vi "GuiderSetupGUI.vi"() -> ()   [LabVIEW 2018]
uses:
  GuiderSetup/GuiderSetup.lvclass
  C:/Users/devstaff/sparc4/s4gui/Versao ZeroMQ REQ-REP/SPARC4_GUI -v1.0.8 - reconhecimento do ACK do ACS/S4GUI/S4GUI.lvclass
  S4GUI/S4GUI.lvclass/S4GUI.ctl
  Instrument/Instrument.lvclass/Instrument.ctl
  Device/Optics/Optics.lvclass/Optics.ctl
  Device/Optics/Opt_Continuous/Opt_Continuous.lvclass
  C:/Users/devstaff/sparc4/s4gui/Versao ZeroMQ REQ-REP/SPARC4_GUI -v1.0.8 - reconhecimento do ACK do ACS/Device/Optics/Optics.lvclass
  Instrument/Instrument.lvclass
  AG/AG.lvclass
  Device/angles/angles.lvclass
  S4GUI/S4GUI.lvclass
  Device/Optics/Optics.lvclass
  StateMachine/State Machine.lvclass
panel:
  out "GUI version":string
  in  "Tab Focus":enum32{"FOCUS", "Config"}(tab)
  in  "Guider Focus Target":dbl caption="Target" min=0.0 max=24.9 step=0.1
  in  "GOTO GFOC":bool
  in  "STOP GFOC":bool
  in  "GFOC IN":bool
  in  "GFOC OUT":bool
  out "Pos GFOC":dbl caption="Position (mm)" format="%3_4g"
  out "GFOC status":bool
  in  "Guider Focus Incr":dbl caption="Increment" min=0.0 max=5.0 step=0.01 format="%#2_4g"
  in  "Set Focus by Mode":bool
  in  "Focus by Mode":T1={"Phot."=17.0, "Polarim"=7.0, "Efficiency"=0.0, "Instrumental"=0.0}
  out "AG connection":bool caption="AG"
  in  "Rotator":dbl caption="ROTATOR"
  out "loop max (ms)":u32
  out "loop time (ms)":u32
  in  "Guider Mirror Veloc":dbl=1.0 caption="Veloc. (1-30)" min=1.0 max=30.0 step=1.0
  out "GMIR status":bool
  out "ICS connection":bool caption="ICS"
  out "error out":errorcluster
  out "Pos GMIR":dbl caption="Position (deg)" format="%-3_4g"
  in  "RUN GMIR":bool
  in  "STOP GMIR":bool
  in  "GOTO GMIR":bool
  in  "Guider Mirror Target":dbl caption="Target"
  in  "stop":bool
  in  "GuiderSetup.lvclass":refnum<class "GuiderSetup.lvclass">
  # "GUIDER SETUP"
  # "MIRROR"
  # "deg"
  # "deg/s"
  # "FOCUS"
  # "mm"
  # "mm"
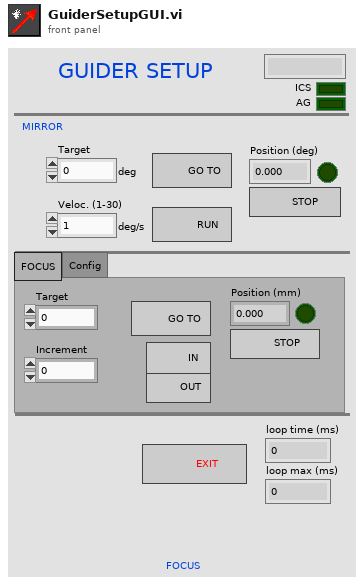
[diagram p1: front panel]
types:
  T1 = cluster{"Phot.":dbl, "Polarim":dbl, "Efficiency":dbl, "Instrumental":dbl}
  T2 = cluster{"Trigger Mode Status":string, "String output":string, "Instrument Status":cluster{"WPROT pos":dbl, "WPSEL pos":dbl, "GMIR pos":dbl, "GFOC pos":dbl, "CALW pos":dbl, "ASEL pos":dbl, "mode":bool, "String Status":string, "connection":bool, "operational":bool}, "Sync Box State":i32, "Trigger General Status":string, "Instrument States":cluster{"WPSEL State":i32, "WPROT State":i32, "CALW State":i32, "ASEL State":i32, "GMIR State":i32, "GFOC State":i32}, "Instrument Pos Names":cluster{"WPROT posname":string, "WPSEL posname":string, "CALW posname":string, "ASEL posname":string}, "ChannelA_Status":cluster{"Current exp":dbl, "Frames done":u32, "LastFileImage":string, "CamStatus":string, "Run state":u32, "connection":bool, "Cooler ON/OFF":i16, "Currently temperature":i16, "Temperature Status":string, "target  temp":i16, "conf runing":bool, "FT":bool, "UsedDisk":u16, "operational":bool}, "WPROT seq":u16, "ChannelB_Status":cluster{"Current exp":dbl, "Frames done":u32, "LastFileImage":string, "CamStatus":string, "Run state":u32, "connection":bool, "Cooler ON/OFF":i16, "Currently temperature":i16, "Temperature Status":string, "target  temp":i16, "conf runing":bool, "FT":bool, "UsedDisk":u16, "operational":bool}, "ChannelC_Status":cluster{"Current exp":dbl, "Frames done":u32, "LastFileImage":string, "CamStatus":string, "Run state":u32, "connection":bool, "Cooler ON/OFF":i16, "Currently temperature":i16, "Temperature Status":string, "target  temp":i16, "conf runing":bool, "FT":bool, "UsedDisk":u16, "operational":bool}, "ChannelD_Status":cluster{"Current exp":dbl, "Frames done":u32, "LastFileImage":string, "CamStatus":string, "Run state":u32, "connection":bool, "Cooler ON/OFF":i16, "Currently temperature":i16, "Temperature Status":string, "target  temp":i16, "conf runing":bool, "FT":bool, "UsedDisk":u16, "operational":bool}, "ChannelA_CCD":cluster{"ACQUISITION_MODE":u8, "TRIGGER_MODE":u8, "READ_MODE":u8, "PREAMP":u8, "READOUT_RATE":u8, "VERTICAL_SHIFT_SPEED":u8, "EM_MODE":u8, "EM_GAIN":u16, "SHUTTER_MODE":u8, "SHUTTER_TTL":u8, "SHUTTER_OPENNING_TIME":u16, "SHUTTER_CLOSING_TIME":u16, "VBIN":u16, "HBIN":u16, "INITIAL_LINE":u16, "INITIAL_COLUMN":u16, "FINAL_LINE":u16, "FINAL_COLUMN":u16, "FRAME_TRANSFER":bool, "VERTICAL_CLOCK_VOLTAGE":u8, "AD_CHANNEL":u32}, "ChannelB_CCD ":cluster{"ACQUISITION_MODE":u8, "TRIGGER_MODE":u8, "READ_MODE":u8, "PREAMP":u8, "READOUT_RATE":u8, "VERTICAL_SHIFT_SPEED":u8, "EM_MODE":u8, "EM_GAIN":u16, "SHUTTER_MODE":u8, "SHUTTER_TTL":u8, "SHUTTER_OPENNING_TIME":u16, "SHUTTER_CLOSING_TIME":u16, "VBIN":u16, "HBIN":u16, "INITIAL_LINE":u16, "INITIAL_COLUMN":u16, "FINAL_LINE":u16, "FINAL_COLUMN":u16, "FRAME_TRANSFER":bool, "VERTICAL_CLOCK_VOLTAGE":u8, "AD_CHANNEL":u32}, "ChannelC_CCD":cluster{"ACQUISITION_MODE":u8, "TRIGGER_MODE":u8, "READ_MODE":u8, "PREAMP":u8, "READOUT_RATE":u8, "VERTICAL_SHIFT_SPEED":u8, "EM_MODE":u8, "EM_GAIN":u16, "SHUTTER_MODE":u8, "SHUTTER_TTL":u8, "SHUTTER_OPENNING_TIME":u16, "SHUTTER_CLOSING_TIME":u16, "VBIN":u16, "HBIN":u16, "INITIAL_LINE":u16, "INITIAL_COLUMN":u16, "FINAL_LINE":u16, "FINAL_COLUMN":u16, "FRAME_TRANSFER":bool, "VERTICAL_CLOCK_VOLTAGE":u8, "AD_CHANNEL":u32}, "ChannelD_CCD":cluster{"ACQUISITION_MODE":u8, "TRIGGER_MODE":u8, "READ_MODE":u8, "PREAMP":u8, "READOUT_RATE":u8, "VERTICAL_SHIFT_SPEED":u8, "EM_MODE":u8, "EM_GAIN":u16, "SHUTTER_MODE":u8, "SHUTTER_TTL":u8, "SHUTTER_OPENNING_TIME":u16, "SHUTTER_CLOSING_TIME":u16, "VBIN":u16, "HBIN":u16, "INITIAL_LINE":u16, "INITIAL_COLUMN":u16, "FINAL_LINE":u16, "FINAL_COLUMN":u16, "FRAME_TRANSFER":bool, "VERTICAL_CLOCK_VOLTAGE":u8, "AD_CHANNEL":u32}, "CHA_Checked Params":cluster{"ACQUISITION_MODE":bool, "TRIGGER_MODE":bool, "READ_MODE":bool, "PREAMP":bool, "READOUT_RATE":bool, "VERTICAL_SHIFT_SPEED":bool, "EM_MODE":bool, "EM_GAIN":bool, "SHUTTER_MODE":bool, "SHUTTER_TTL":bool, "SHUTTER_OPENING_TIME":bool, "SHUTTER_CLOSING_TIME":bool, "VBIN":bool, "HBIN":bool, "INITIAL_LINE":bool, "INITIAL_COLUMN":bool, "FINAL_LINE":bool, "FINAL_COLUMN":bool, "FRAME_TRANSFER":bool, "VERTICAL_CLOCK_VOLTAGE":bool, "AD_CHANNEL":bool}, "CHB_Checked Params":cluster{"ACQUISITION_MODE":bool, "TRIGGER_MODE":bool, "READ_MODE":bool, "PREAMP":bool, "READOUT_RATE":bool, "VERTICAL_SHIFT_SPEED":bool, "EM_MODE":bool, "EM_GAIN":bool, "SHUTTER_MODE":bool, "SHUTTER_TTL":bool, "SHUTTER_OPENING_TIME":bool, "SHUTTER_CLOSING_TIME":bool, "VBIN":bool, "HBIN":bool, "INITIAL_LINE":bool, "INITIAL_COLUMN":bool, "FINAL_LINE":bool, "FINAL_COLUMN":bool, "FRAME_TRANSFER":bool, "VERTICAL_CLOCK_VOLTAGE":bool, "AD_CHANNEL":bool}, "CHC_Checked Params":cluster{"ACQUISITION_MODE":bool, "TRIGGER_MODE":bool, "READ_MODE":bool, "PREAMP":bool, "READOUT_RATE":bool, "VERTICAL_SHIFT_SPEED":bool, "EM_MODE":bool, "EM_GAIN":bool, "SHUTTER_MODE":bool, "SHUTTER_TTL":bool, "SHUTTER_OPENING_TIME":bool, "SHUTTER_CLOSING_TIME":bool, "VBIN":bool, "HBIN":bool, "INITIAL_LINE":bool, "INITIAL_COLUMN":bool, "FINAL_LINE":bool, "FINAL_COLUMN":bool, "FRAME_TRANSFER":bool, "VERTICAL_CLOCK_VOLTAGE":bool, "AD_CHANNEL":bool}, "CHD_Checked Params":cluster{"ACQUISITION_MODE":bool, "TRIGGER_MODE":bool, "READ_MODE":bool, "PREAMP":bool, "READOUT_RATE":bool, "VERTICAL_SHIFT_SPEED":bool, "EM_MODE":bool, "EM_GAIN":bool, "SHUTTER_MODE":bool, "SHUTTER_TTL":bool, "SHUTTER_OPENING_TIME":bool, "SHUTTER_CLOSING_TIME":bool, "VBIN":bool, "HBIN":bool, "INITIAL_LINE":bool, "INITIAL_COLUMN":bool, "FINAL_LINE":bool, "FINAL_COLUMN":bool, "FRAME_TRANSFER":bool, "VERTICAL_CLOCK_VOLTAGE":bool, "AD_CHANNEL":bool}, "Trigger_connection":bool, "TCSPD_connection":bool, "TCS extended":string, "TCS id":u32, "S4ICS id":u32, "focus pos":i32, "Focus_connection":bool, "WS_connection":bool, "weather status":cluster{"broker":string, "version":string, "date":string, "hour":string, "outHumidity":string, "inHumidity":string, "inTemp":string, "outTemp":string, "windSpeed":string, "windDirection":string, "pressure":string, "dewOut":string, "dewIn":string, "leaf":string, "rain":string, "windChill":string}, "GS STATUS cluster":cluster{"FocusPhot":dbl, "FocusPolar":dbl, "FocusEffic":dbl, "FocusInstrum":dbl, "ICS":bool, "AG":bool, "BROKER":string, "timestamp":string, "FocusPos":dbl, "MirrorPos":dbl}, "TCSPD_operational":bool, "Focus_operational":bool, "object_suffix":string, "dflat_suffix":string, "sflat_suffix":string, "dark_suffix":string, "zero_suffix":string, "focus_suffix":string, "suffixAlertVisible":bool, "Instrument Motor error":cluster{"WPSEL error":bool, "WPROT error":bool, "CALW error":bool, "ASEL error":bool, "GMIR error":bool, "GFOC error":bool}}
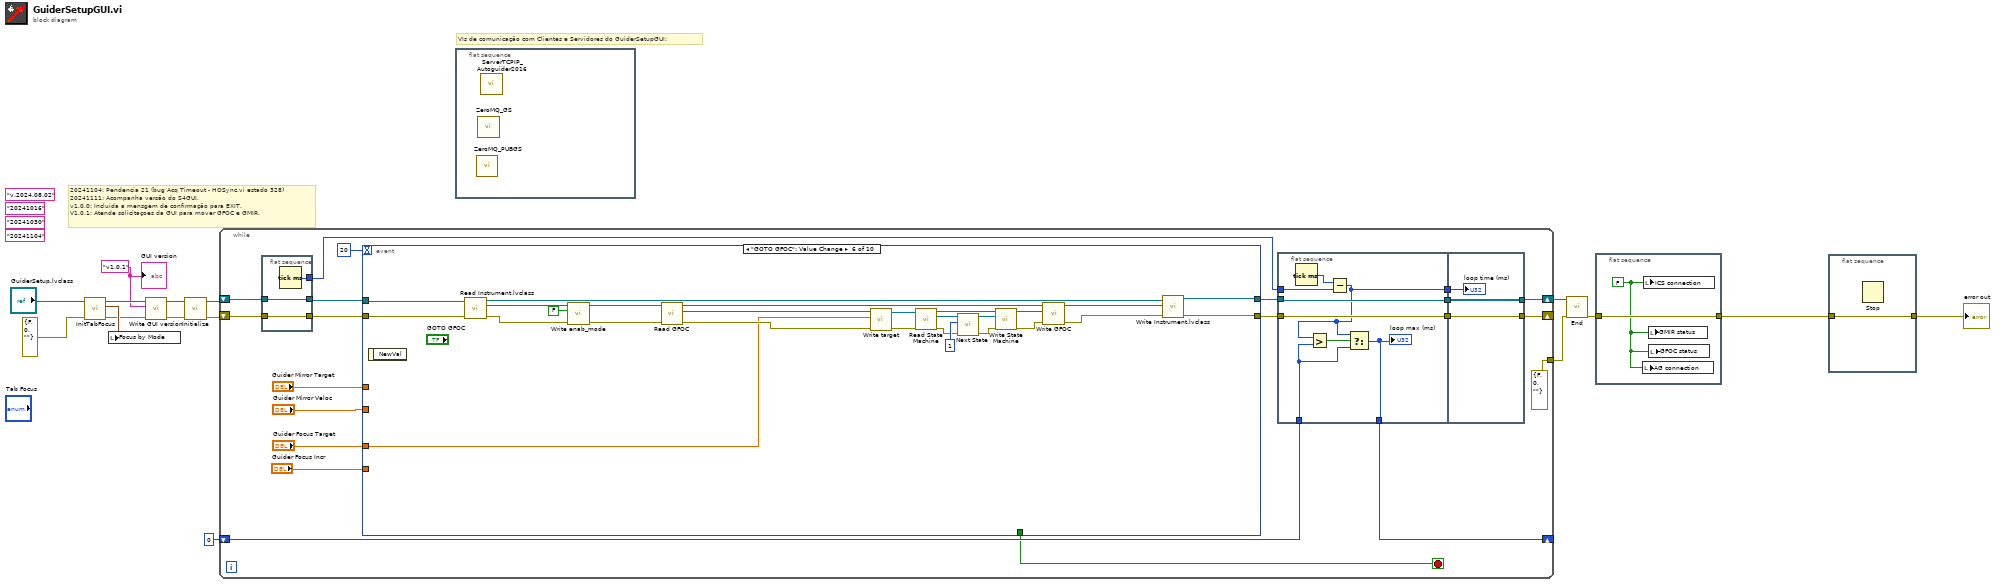
[diagram p0: block diagram]
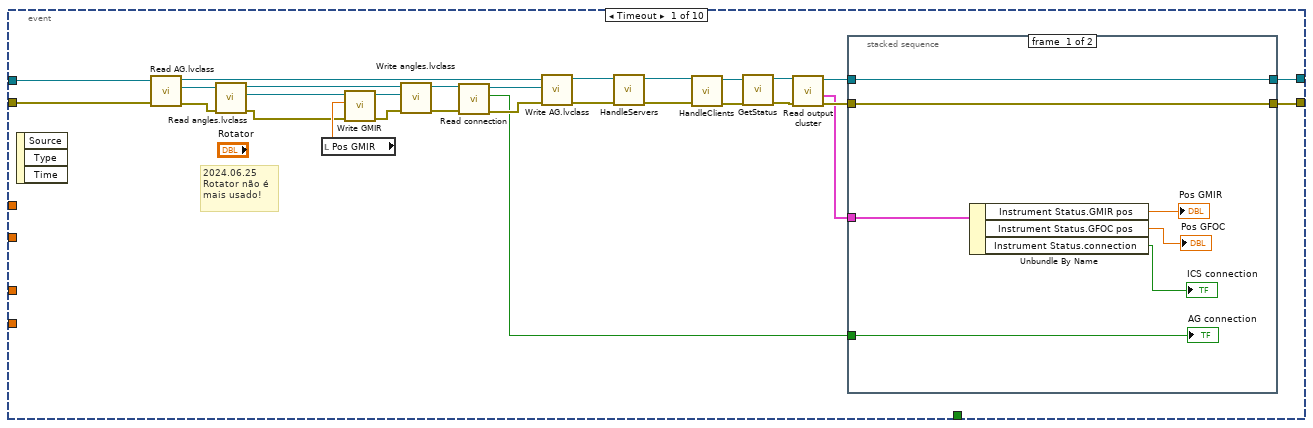
[diagram p2: hidden frame]
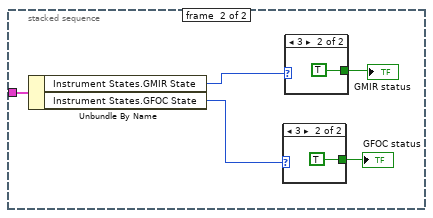
[diagram p3: hidden frame]
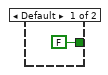
[diagram p4: hidden frame]
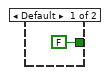
[diagram p5: hidden frame]
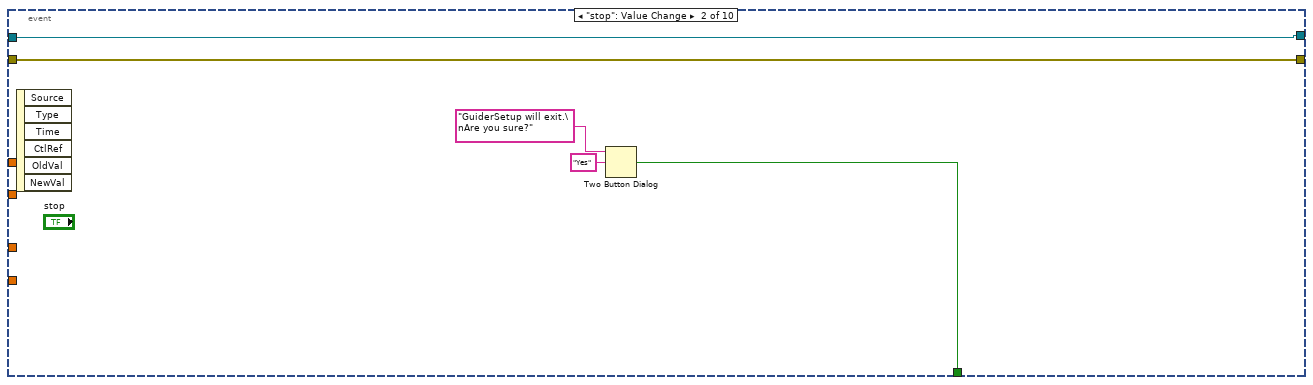
[diagram p6: hidden frame]
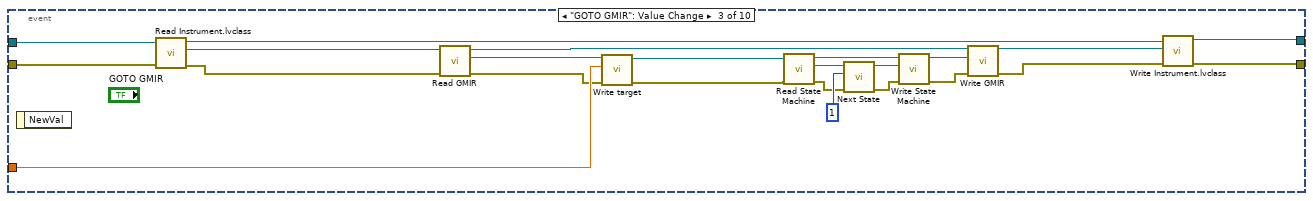
[diagram p7: hidden frame]
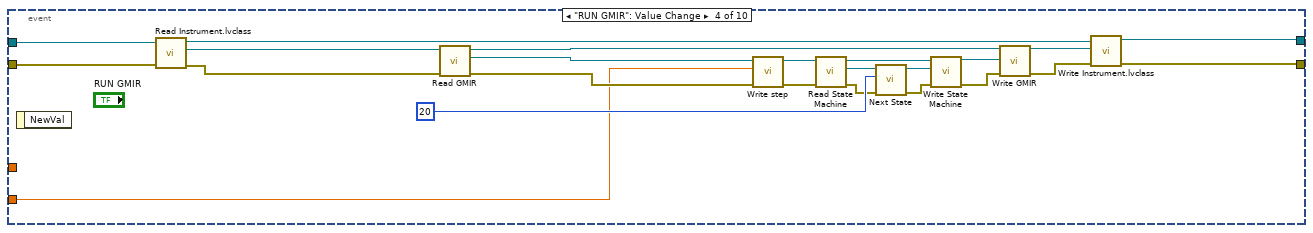
[diagram p8: hidden frame]
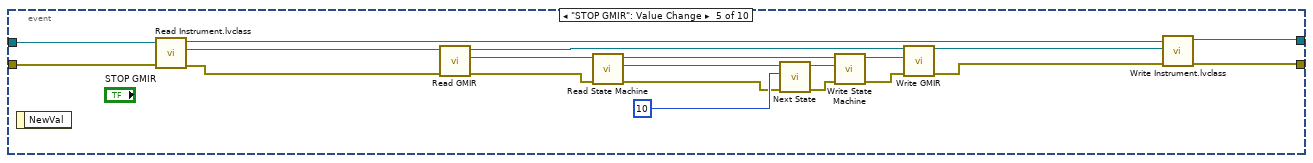
[diagram p9: hidden frame]
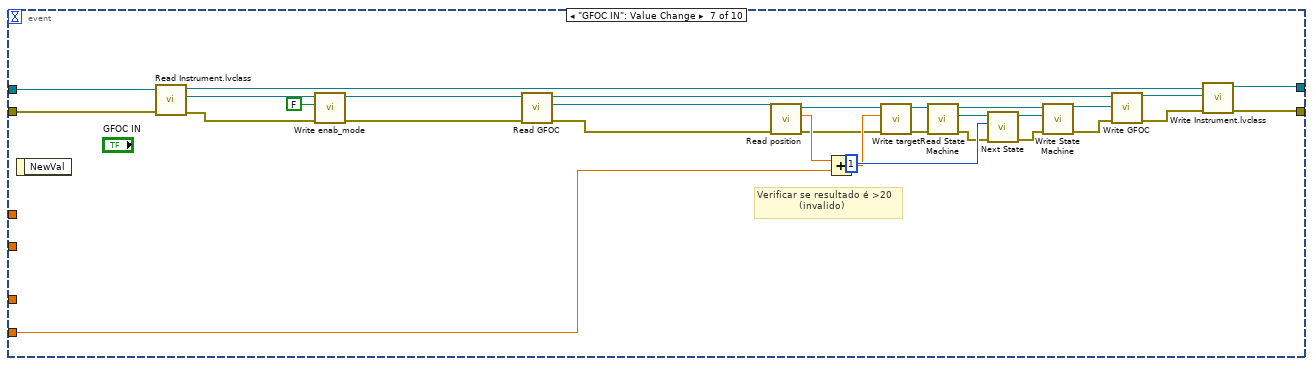
[diagram p10: hidden frame]
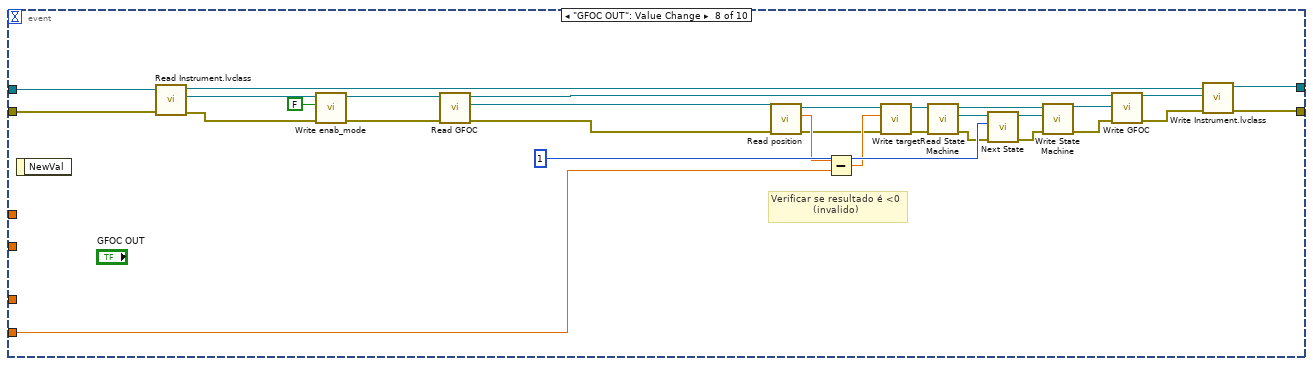
[diagram p11: hidden frame]
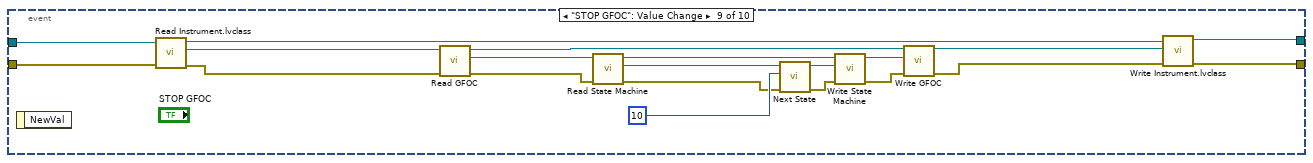
[diagram p12: hidden frame]
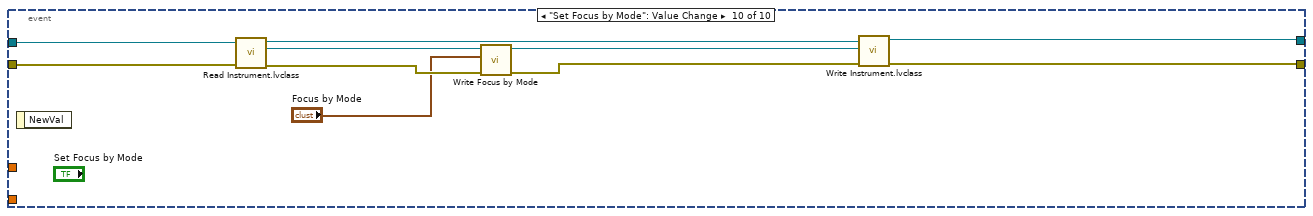
[diagram p13: hidden frame]
diagram:
  (unwired) "20241104" ("GUI version")
  (unwired) "20241030" ("GUI version")
  (unwired) "20241016" ("GUI version")
  w1 = "v1.0.1" ("GUI version")
  (unwired) "v.2024.08.02" ("GUI version")
  # "20241104: Pendencia 21 (bug Acq Timeout - HOSync.vi estado 328)\n20241111: Acompanha versão do S4GUI.\nv1.0.0: Incluída a mensgem de confirmação para EXIT.\nV1.0.1: Atende solicitaçoes da GUI para mover GFOC e GMIR."
  # "VIs de comunicação com Clientes e Servidores do GuiderSetupGUI:"
  n1 = call-dynamic "InitTabFocus.vi"("error in (no error)"=errorcluster {"status"=FALSE, "code"=0, "source"=""}, "GuiderSetup in"="GuiderSetup.lvclass") -> ("error out"=w5:errorcluster, "output cluster"=w8:T1, "GuiderSetup out"=w7:refnum<class "GuiderSetup.lvclass">)  [unwired: 7 in]
  n2 = local write "Focus by Mode"(w8) -> ()
  n3 = call-dynamic "Write GUI version.vi"("error in (no error)"=w5, "GUI version"=w1, "S4GUI in"=w7) -> ("error out"=w4:errorcluster, "S4GUI out"=w6:refnum<class "GuiderSetup.lvclass">)  [unwired: 7 in]
  n4 = call-dynamic "Initialize.vi"("error in (no error)"=w4, "S4ACS_GUI in"=w6) -> ("error out"=w15:errorcluster, "S4ACS_GUI out"=w16:refnum<class "GuiderSetup.lvclass">)  [unwired: 8 in]
  n5 = while {
    shift-right: [w25] -> w14
    shift-left: w16 -> [w32]
    shift-right: [w26] -> _
    shift-left: w15 -> [w31]
    shift-right: [w20] -> _
    shift-left: u32 0 -> [w19]
    tunnel: [errorcluster {"status"=FALSE, "code"=0, "source"=""} ("error in (no error)")] -> w11
    stop <- w17 stop-if-true
    n6 = flat-sequence {
      tunnel: [w51] -> w21
      tunnel: w32 -> [w50]
      tunnel: w31 -> [w49]
      tunnel: [w50] -> w30
      tunnel: [w49] -> w29
      frame #0 {
        n7 = Tick Count (ms)() -> (millisecond timer value=w51:u32)
      }
    }
    n8 = event shown="[5] \"GOTO GFOC\": Value Change" {
      selector: _ -> [_ _ _ _ _ _ _ _ _ _]
      dyn-events: _ -> [_ _ _ _ _ _ _ _ _ _]
      timeout: 20 -> [_ _ _ _ _ _ _ _ _ _]
      tunnel: w30 -> [w80 w101 w124 w147 w167 w193 w223 w253 w273 w283]
      tunnel: [w64 w101 w122 w145 w165 w191 w221 w251 w271 w281] -> w28
      tunnel: w29 -> [w79 w98 w118 w141 w161 w188 w218 w248 w267 w280]
      tunnel: [w61 w98 w115 w138 w158 w186 w216 w246 w264 w279] -> w27
      tunnel: "Guider Mirror Veloc" -> [_ _ _ w125 _ _ _ _ _ _]
      tunnel: "Guider Mirror Target" -> [_ _ w104 _ _ _ _ _ _ _]
      tunnel: "Guider Focus Target" -> [_ _ _ _ _ w173 _ _ _ _]
      tunnel: "Guider Focus Incr" -> [_ _ _ _ _ _ w199 w229 _ _]
      tunnel: [_ w99 _ _ _ _ _ _ _ _] -> w17
      event Timeout {
        # "2024.06.25\nRotator não é \nmais usado!"
        n9 = event-data() -> ()  [unwired: 1 in, 3 out]
        n10 = call-dynamic "Read AG.lvclass.vi"("error in (no error)"=w79, "GuiderSetup in"=w80) -> ("error out"=w74:errorcluster, "AG.lvclass"=w77:refnum<class "AG.lvclass">, "GuiderSetup out"=w78:refnum<class "GuiderSetup.lvclass">)  [unwired: 7 in]
        n11 = call-dynamic "Read angles.lvclass.vi"("error in (no error)"=w74, "AG in"=w77) -> ("error out"=w62:errorcluster, "angles.lvclass"=w63:refnum<class "angles.lvclass">, "AG out"=w76:refnum<class "AG.lvclass">)  [unwired: 7 in]
        n12 = local read "Pos GMIR"() -> (w72:dbl)
        n13 = call-dynamic "Write GMIR.vi"("error in (no error)"=w62, "GMIR"=w72, "angles in"=w63) -> ("error out"=w73:errorcluster, "angles out"=w75:refnum<class "angles.lvclass">)  [unwired: 7 in]
        n14 = call-dynamic "Write angles.lvclass.vi"("error in (no error)"=w73, "angles.lvclass"=w75, "AG in"=w76) -> ("error out"=w67:errorcluster, "AG out"=w69:refnum<class "AG.lvclass">)  [unwired: 7 in]
        n15 = call-dynamic "Read connection.vi"("error in (no error)"=w67, "Client in"=w69) -> ("error out"=w66:errorcluster, "connection"=w65:bool, "Client out"=w68:refnum<class "AG.lvclass">)  [unwired: 7 in]
        n16 = call-dynamic "Write AG.lvclass.vi"("error in (no error)"=w66, "AG.lvclass"=w68, "GuiderSetup in"=w78) -> ("error out"=w71:errorcluster, "GuiderSetup out"=w70:refnum<class "GuiderSetup.lvclass">)  [unwired: 7 in]
        n17 = call-dynamic "HandleServers.vi"("error in (no error)"=w71, "S4ACS_GUI in"=w70) -> ("error out"=w58:errorcluster, "S4ACS_GUI out"=w60:refnum<class "GuiderSetup.lvclass">)  [unwired: 8 in]
        n18 = call-dynamic "HandleClients.vi"("error in (no error)"=w58, "GuiderSetup in"=w60) -> ("error out"=w57:errorcluster, "GuiderSetup out"=w59:refnum<class "GuiderSetup.lvclass">)  [unwired: 8 in]
        n19 = call-dynamic "GetStatus.vi"("error in (no error)"=w57, "GS in"=w59) -> ("error out"=w54:errorcluster, "GS out"=w56:refnum<class "GuiderSetup.lvclass">)  [unwired: 8 in]
        n20 = call-dynamic "Read output cluster.vi"("error in (no error)"=w54, "S4GUI in"=w56) -> ("error out"=w53:errorcluster, "output cluster"=w52:T2, "S4GUI out"=w55:refnum<class "GuiderSetup.lvclass">)  [unwired: 7 in]
        n21 = stacked-sequence {
          tunnel: w65 -> [w84 _]
          tunnel: w55 -> [w83 _]
          tunnel: w53 -> [w82 _]
          tunnel: [w83 _] -> w64
          tunnel: [w82 _] -> w61
          tunnel: w52 -> [w81 w88]
          frame #0 {
            n22 = Unbundle By Name(w81) -> ("Instrument Status.GMIR pos"=→"Pos GMIR":dbl, "Instrument Status.GFOC pos"=→"Pos GFOC":dbl, "Instrument Status.connection"=→"ICS connection":bool)
            "AG connection" <- w84
          }
          frame #1 {
            n23 = Unbundle By Name(w88) -> ("Instrument States.GMIR State"=w92:i32, "Instrument States.GFOC State"=w90:i32)
            n24 = case shown="3" w90 {
              tunnel: [FALSE TRUE] -> w89
              frame Default {
              }
              frame 3 {
              }
            }
            "GFOC status" <- w89
            n25 = case shown="3" w92 {
              tunnel: [FALSE TRUE] -> w91
              frame Default {
              }
              frame 3 {
              }
            }
            "GMIR status" <- w91
          }
        }
      }
      event "stop": Value Change {
        n26 = event-data() -> ()  [unwired: 1 in, 6 out]
        n27 = Two Button Dialog(message="GuiderSetup will exit.\nAre you sure?", 2:"Yes" ("T button name (\"OK\")")) -> (T button?=w99:bool)  [unwired: 1 in]
      }
      event "GOTO GMIR": Value Change {
        n28 = event-data() -> ()  [unwired: 1 in, 1 out]
        n29 = call "Read Instrument.lvclass.vi"("error in (no error)"=w118, "S4ACS_GUI in"=w124) -> ("error out"=w117:errorcluster, "Instrument.lvclass"=w121:refnum<class "Instrument.lvclass">, "S4ACS_GUI out"=w123:refnum<class "GuiderSetup.lvclass">)  [unwired: 7 in]
        n30 = call "Read GMIR.vi"("error in (no error)"=w117, "Instrument in"=w121) -> ("error out"=w103:errorcluster, "Opt_Continuous.lvclass"=w106:refnum<class "Opt_Continuous.lvclass">, "Instrument out"=w120:refnum<class "Instrument.lvclass">)  [unwired: 7 in]
        n31 = call "Write target.vi"("error in (no error)"=w103, "target"=w104, "Optics in"=w106) -> ("error out"=w102:errorcluster, "Optics out"=w105:refnum<class "Opt_Continuous.lvclass">)  [unwired: 7 in]
        n32 = call-dynamic "Read State Machine.vi"("error in (no error)"=w102, "Device in"=w105) -> ("error out"=w109:errorcluster, "State Machine.lvclass"=w112:refnum<class "State Machine.lvclass">, "Device out"=w114:refnum<class "Opt_Continuous.lvclass">)  [unwired: 7 in]
        n33 = call "Next State.vi"("error in (no error)"=w109, "New_State"=1, "State Machine in"=w112) -> ("error out"=w108:errorcluster, "State Machine out"=w111:refnum<class "State Machine.lvclass">)  [unwired: 7 in]
        n34 = call-dynamic "Write State Machine.vi"("error in (no error)"=w108, "State Machine.lvclass"=w111, "Device in"=w114) -> ("error out"=w107:errorcluster, "Device out"=w113:refnum<class "Opt_Continuous.lvclass">)  [unwired: 7 in]
        n35 = call "Write GMIR.vi"("error in (no error)"=w107, "Opt_Continuous.lvclass"=w113, "Instrument in"=w120) -> ("error out"=w116:errorcluster, "Instrument out"=w119:refnum<class "Instrument.lvclass">)  [unwired: 7 in]
        n36 = call "Write Instrument.lvclass.vi"("error in (no error)"=w116, "Instrument.lvclass"=w119, "S4ACS_GUI in"=w123) -> ("error out"=w115:errorcluster, "S4ACS_GUI out"=w122:refnum<class "GuiderSetup.lvclass">)  [unwired: 7 in]
      }
      event "RUN GMIR": Value Change {
        n37 = event-data() -> ()  [unwired: 1 in, 1 out]
        n38 = call "Read Instrument.lvclass.vi"("error in (no error)"=w141, "S4ACS_GUI in"=w147) -> ("error out"=w140:errorcluster, "Instrument.lvclass"=w144:refnum<class "Instrument.lvclass">, "S4ACS_GUI out"=w146:refnum<class "GuiderSetup.lvclass">)  [unwired: 7 in]
        n39 = call "Read GMIR.vi"("error in (no error)"=w140, "Instrument in"=w144) -> ("error out"=w128:errorcluster, "Opt_Continuous.lvclass"=w129:refnum<class "Opt_Continuous.lvclass">, "Instrument out"=w143:refnum<class "Instrument.lvclass">)  [unwired: 7 in]
        n40 = call-dynamic "Write step.vi"("error in (no error)"=w128, "step"=w125, "Optics in"=w129) -> ("error out"=w127:errorcluster, "Optics out"=w126:refnum<class "Opt_Continuous.lvclass">)  [unwired: 7 in]
        n41 = call-dynamic "Read State Machine.vi"("error in (no error)"=w127, "Device in"=w126) -> ("error out"=w132:errorcluster, "State Machine.lvclass"=w135:refnum<class "State Machine.lvclass">, "Device out"=w137:refnum<class "Opt_Continuous.lvclass">)  [unwired: 7 in]
        n42 = call "Next State.vi"("error in (no error)"=w132, "New_State"=20, "State Machine in"=w135) -> ("error out"=w131:errorcluster, "State Machine out"=w134:refnum<class "State Machine.lvclass">)  [unwired: 7 in]
        n43 = call-dynamic "Write State Machine.vi"("error in (no error)"=w131, "State Machine.lvclass"=w134, "Device in"=w137) -> ("error out"=w130:errorcluster, "Device out"=w136:refnum<class "Opt_Continuous.lvclass">)  [unwired: 7 in]
        n44 = call "Write GMIR.vi"("error in (no error)"=w130, "Opt_Continuous.lvclass"=w136, "Instrument in"=w143) -> ("error out"=w139:errorcluster, "Instrument out"=w142:refnum<class "Instrument.lvclass">)  [unwired: 7 in]
        n45 = call "Write Instrument.lvclass.vi"("error in (no error)"=w139, "Instrument.lvclass"=w142, "S4ACS_GUI in"=w146) -> ("error out"=w138:errorcluster, "S4ACS_GUI out"=w145:refnum<class "GuiderSetup.lvclass">)  [unwired: 7 in]
      }
      event "STOP GMIR": Value Change {
        n46 = event-data() -> ()  [unwired: 1 in, 1 out]
        n47 = call "Read Instrument.lvclass.vi"("error in (no error)"=w161, "S4ACS_GUI in"=w167) -> ("error out"=w160:errorcluster, "Instrument.lvclass"=w164:refnum<class "Instrument.lvclass">, "S4ACS_GUI out"=w166:refnum<class "GuiderSetup.lvclass">)  [unwired: 7 in]
        n48 = call "Read GMIR.vi"("error in (no error)"=w160, "Instrument in"=w164) -> ("error out"=w151:errorcluster, "Opt_Continuous.lvclass"=w157:refnum<class "Opt_Continuous.lvclass">, "Instrument out"=w163:refnum<class "Instrument.lvclass">)  [unwired: 7 in]
        n49 = call-dynamic "Read State Machine.vi"("error in (no error)"=w151, "Device in"=w157) -> ("error out"=w150:errorcluster, "State Machine.lvclass"=w154:refnum<class "State Machine.lvclass">, "Device out"=w156:refnum<class "Opt_Continuous.lvclass">)  [unwired: 7 in]
        n50 = call "Next State.vi"("error in (no error)"=w150, "New_State"=10, "State Machine in"=w154) -> ("error out"=w149:errorcluster, "State Machine out"=w153:refnum<class "State Machine.lvclass">)  [unwired: 7 in]
        n51 = call-dynamic "Write State Machine.vi"("error in (no error)"=w149, "State Machine.lvclass"=w153, "Device in"=w156) -> ("error out"=w148:errorcluster, "Device out"=w155:refnum<class "Opt_Continuous.lvclass">)  [unwired: 7 in]
        n52 = call "Write GMIR.vi"("error in (no error)"=w148, "Opt_Continuous.lvclass"=w155, "Instrument in"=w163) -> ("error out"=w159:errorcluster, "Instrument out"=w162:refnum<class "Instrument.lvclass">)  [unwired: 7 in]
        n53 = call "Write Instrument.lvclass.vi"("error in (no error)"=w159, "Instrument.lvclass"=w162, "S4ACS_GUI in"=w166) -> ("error out"=w158:errorcluster, "S4ACS_GUI out"=w165:refnum<class "GuiderSetup.lvclass">)  [unwired: 7 in]
      }
      event "GOTO GFOC": Value Change {
        n54 = event-data() -> ()  [unwired: 1 in, 1 out]
        n55 = call "Read Instrument.lvclass.vi"("error in (no error)"=w188, "S4ACS_GUI in"=w193) -> ("error out"=w171:errorcluster, "Instrument.lvclass"=w172:refnum<class "Instrument.lvclass">, "S4ACS_GUI out"=w192:refnum<class "GuiderSetup.lvclass">)  [unwired: 7 in]
        n56 = call-dynamic "Write enab_mode.vi"("error in (no error)"=w171, "enab_mode"=FALSE, "Instrument in"=w172) -> ("error out"=w168:errorcluster, "Instrument out"=w169:refnum<class "Instrument.lvclass">)  [unwired: 7 in]
        n57 = call "Read GFOC.vi"("error in (no error)"=w168, "Instrument in"=w169) -> ("error out"=w175:errorcluster, "Opt_Continuous.lvclass"=w177:refnum<class "Opt_Continuous.lvclass">, "Instrument out"=w190:refnum<class "Instrument.lvclass">)  [unwired: 7 in]
        n58 = call "Write target.vi"("error in (no error)"=w175, "target"=w173, "Optics in"=w177) -> ("error out"=w174:errorcluster, "Optics out"=w176:refnum<class "Opt_Continuous.lvclass">)  [unwired: 7 in]
        n59 = call-dynamic "Read State Machine.vi"("error in (no error)"=w174, "Device in"=w176) -> ("error out"=w180:errorcluster, "State Machine.lvclass"=w183:refnum<class "State Machine.lvclass">, "Device out"=w185:refnum<class "Opt_Continuous.lvclass">)  [unwired: 7 in]
        n60 = call "Next State.vi"("error in (no error)"=w180, "New_State"=1, "State Machine in"=w183) -> ("error out"=w179:errorcluster, "State Machine out"=w182:refnum<class "State Machine.lvclass">)  [unwired: 7 in]
        n61 = call-dynamic "Write State Machine.vi"("error in (no error)"=w179, "State Machine.lvclass"=w182, "Device in"=w185) -> ("error out"=w178:errorcluster, "Device out"=w184:refnum<class "Opt_Continuous.lvclass">)  [unwired: 7 in]
        n62 = call "Write GFOC.vi"("error in (no error)"=w178, "Opt_Continuous.lvclass"=w184, "Instrument in"=w190) -> ("error out"=w187:errorcluster, "Instrument out"=w189:refnum<class "Instrument.lvclass">)  [unwired: 7 in]
        n63 = call "Write Instrument.lvclass.vi"("error in (no error)"=w187, "Instrument.lvclass"=w189, "S4ACS_GUI in"=w192) -> ("error out"=w186:errorcluster, "S4ACS_GUI out"=w191:refnum<class "GuiderSetup.lvclass">)  [unwired: 7 in]
      }
      event "GFOC IN": Value Change {
        # "Verificar se resultado é >20 \n              (invalido)"
        n64 = event-data() -> ()  [unwired: 1 in, 1 out]
        n65 = call "Read Instrument.lvclass.vi"("error in (no error)"=w218, "S4ACS_GUI in"=w223) -> ("error out"=w196:errorcluster, "Instrument.lvclass"=w197:refnum<class "Instrument.lvclass">, "S4ACS_GUI out"=w222:refnum<class "GuiderSetup.lvclass">)  [unwired: 7 in]
        n66 = call-dynamic "Write enab_mode.vi"("error in (no error)"=w196, "enab_mode"=FALSE, "Instrument in"=w197) -> ("error out"=w194:errorcluster, "Instrument out"=w195:refnum<class "Instrument.lvclass">)  [unwired: 7 in]
        n67 = call "Read GFOC.vi"("error in (no error)"=w194, "Instrument in"=w195) -> ("error out"=w200:errorcluster, "Opt_Continuous.lvclass"=w201:refnum<class "Opt_Continuous.lvclass">, "Instrument out"=w220:refnum<class "Instrument.lvclass">)  [unwired: 7 in]
        n68 = call "Read position.vi"("error in (no error)"=w200, "Optics in"=w201) -> ("error out"=w204:errorcluster, "position"=w207:dbl, "Optics out"=w205:refnum<class "Opt_Continuous.lvclass">)  [unwired: 7 in]
        n69 = Add(x=w207, y=w199) -> (x+y=w206:dbl)
        n70 = call "Write target.vi"("error in (no error)"=w204, "target"=w206, "Optics in"=w205) -> ("error out"=w203:errorcluster, "Optics out"=w202:refnum<class "Opt_Continuous.lvclass">)  [unwired: 7 in]
        n71 = call-dynamic "Read State Machine.vi"("error in (no error)"=w203, "Device in"=w202) -> ("error out"=w210:errorcluster, "State Machine.lvclass"=w213:refnum<class "State Machine.lvclass">, "Device out"=w215:refnum<class "Opt_Continuous.lvclass">)  [unwired: 7 in]
        n72 = call "Next State.vi"("error in (no error)"=w210, "New_State"=1, "State Machine in"=w213) -> ("error out"=w209:errorcluster, "State Machine out"=w212:refnum<class "State Machine.lvclass">)  [unwired: 7 in]
        n73 = call-dynamic "Write State Machine.vi"("error in (no error)"=w209, "State Machine.lvclass"=w212, "Device in"=w215) -> ("error out"=w208:errorcluster, "Device out"=w214:refnum<class "Opt_Continuous.lvclass">)  [unwired: 7 in]
        n74 = call "Write GFOC.vi"("error in (no error)"=w208, "Opt_Continuous.lvclass"=w214, "Instrument in"=w220) -> ("error out"=w217:errorcluster, "Instrument out"=w219:refnum<class "Instrument.lvclass">)  [unwired: 7 in]
        n75 = call "Write Instrument.lvclass.vi"("error in (no error)"=w217, "Instrument.lvclass"=w219, "S4ACS_GUI in"=w222) -> ("error out"=w216:errorcluster, "S4ACS_GUI out"=w221:refnum<class "GuiderSetup.lvclass">)  [unwired: 7 in]
      }
      event "GFOC OUT": Value Change {
        # "Verificar se resultado é <0\n              (invalido)"
        n76 = event-data() -> ()  [unwired: 1 in, 1 out]
        n77 = call "Read Instrument.lvclass.vi"("error in (no error)"=w248, "S4ACS_GUI in"=w253) -> ("error out"=w226:errorcluster, "Instrument.lvclass"=w227:refnum<class "Instrument.lvclass">, "S4ACS_GUI out"=w252:refnum<class "GuiderSetup.lvclass">)  [unwired: 7 in]
        n78 = call-dynamic "Write enab_mode.vi"("error in (no error)"=w226, "enab_mode"=FALSE, "Instrument in"=w227) -> ("error out"=w224:errorcluster, "Instrument out"=w225:refnum<class "Instrument.lvclass">)  [unwired: 7 in]
        n79 = call "Read GFOC.vi"("error in (no error)"=w224, "Instrument in"=w225) -> ("error out"=w230:errorcluster, "Opt_Continuous.lvclass"=w231:refnum<class "Opt_Continuous.lvclass">, "Instrument out"=w250:refnum<class "Instrument.lvclass">)  [unwired: 7 in]
        n80 = call "Read position.vi"("error in (no error)"=w230, "Optics in"=w231) -> ("error out"=w234:errorcluster, "position"=w237:dbl, "Optics out"=w235:refnum<class "Opt_Continuous.lvclass">)  [unwired: 7 in]
        n81 = Subtract(x=w237, y=w229) -> (x-y=w236:dbl)
        n82 = call "Write target.vi"("error in (no error)"=w234, "target"=w236, "Optics in"=w235) -> ("error out"=w233:errorcluster, "Optics out"=w232:refnum<class "Opt_Continuous.lvclass">)  [unwired: 7 in]
        n83 = call-dynamic "Read State Machine.vi"("error in (no error)"=w233, "Device in"=w232) -> ("error out"=w240:errorcluster, "State Machine.lvclass"=w243:refnum<class "State Machine.lvclass">, "Device out"=w245:refnum<class "Opt_Continuous.lvclass">)  [unwired: 7 in]
        n84 = call "Next State.vi"("error in (no error)"=w240, "New_State"=1, "State Machine in"=w243) -> ("error out"=w239:errorcluster, "State Machine out"=w242:refnum<class "State Machine.lvclass">)  [unwired: 7 in]
        n85 = call-dynamic "Write State Machine.vi"("error in (no error)"=w239, "State Machine.lvclass"=w242, "Device in"=w245) -> ("error out"=w238:errorcluster, "Device out"=w244:refnum<class "Opt_Continuous.lvclass">)  [unwired: 7 in]
        n86 = call "Write GFOC.vi"("error in (no error)"=w238, "Opt_Continuous.lvclass"=w244, "Instrument in"=w250) -> ("error out"=w247:errorcluster, "Instrument out"=w249:refnum<class "Instrument.lvclass">)  [unwired: 7 in]
        n87 = call "Write Instrument.lvclass.vi"("error in (no error)"=w247, "Instrument.lvclass"=w249, "S4ACS_GUI in"=w252) -> ("error out"=w246:errorcluster, "S4ACS_GUI out"=w251:refnum<class "GuiderSetup.lvclass">)  [unwired: 7 in]
      }
      event "STOP GFOC": Value Change {
        n88 = event-data() -> ()  [unwired: 1 in, 1 out]
        n89 = call "Read Instrument.lvclass.vi"("error in (no error)"=w267, "S4ACS_GUI in"=w273) -> ("error out"=w266:errorcluster, "Instrument.lvclass"=w270:refnum<class "Instrument.lvclass">, "S4ACS_GUI out"=w272:refnum<class "GuiderSetup.lvclass">)  [unwired: 7 in]
        n90 = call "Read GFOC.vi"("error in (no error)"=w266, "Instrument in"=w270) -> ("error out"=w257:errorcluster, "Opt_Continuous.lvclass"=w263:refnum<class "Opt_Continuous.lvclass">, "Instrument out"=w269:refnum<class "Instrument.lvclass">)  [unwired: 7 in]
        n91 = call-dynamic "Read State Machine.vi"("error in (no error)"=w257, "Device in"=w263) -> ("error out"=w256:errorcluster, "State Machine.lvclass"=w260:refnum<class "State Machine.lvclass">, "Device out"=w262:refnum<class "Opt_Continuous.lvclass">)  [unwired: 7 in]
        n92 = call "Next State.vi"("error in (no error)"=w256, "New_State"=10, "State Machine in"=w260) -> ("error out"=w255:errorcluster, "State Machine out"=w259:refnum<class "State Machine.lvclass">)  [unwired: 7 in]
        n93 = call-dynamic "Write State Machine.vi"("error in (no error)"=w255, "State Machine.lvclass"=w259, "Device in"=w262) -> ("error out"=w254:errorcluster, "Device out"=w261:refnum<class "Opt_Continuous.lvclass">)  [unwired: 7 in]
        n94 = call "Write GFOC.vi"("error in (no error)"=w254, "Opt_Continuous.lvclass"=w261, "Instrument in"=w269) -> ("error out"=w265:errorcluster, "Instrument out"=w268:refnum<class "Instrument.lvclass">)  [unwired: 7 in]
        n95 = call "Write Instrument.lvclass.vi"("error in (no error)"=w265, "Instrument.lvclass"=w268, "S4ACS_GUI in"=w272) -> ("error out"=w264:errorcluster, "S4ACS_GUI out"=w271:refnum<class "GuiderSetup.lvclass">)  [unwired: 7 in]
      }
      event "Set Focus by Mode": Value Change {
        n96 = event-data() -> ()  [unwired: 1 in, 1 out]
        n97 = call "Read Instrument.lvclass.vi"("error in (no error)"=w280, "S4ACS_GUI in"=w283) -> ("error out"=w277:errorcluster, "Instrument.lvclass"=w278:refnum<class "Instrument.lvclass">, "S4ACS_GUI out"=w282:refnum<class "GuiderSetup.lvclass">)  [unwired: 7 in]
        n98 = call-dynamic "Write Focus by Mode.vi"("error in (no error)"=w277, "Focus by Mode"="Focus by Mode", "Instrument in"=w278) -> ("error out"=w275:errorcluster, "Instrument out"=w276:refnum<class "Instrument.lvclass">)  [unwired: 7 in]
        n99 = call "Write Instrument.lvclass.vi"("error in (no error)"=w275, "Instrument.lvclass"=w276, "S4ACS_GUI in"=w282) -> ("error out"=w279:errorcluster, "S4ACS_GUI out"=w281:refnum<class "GuiderSetup.lvclass">)  [unwired: 7 in]
      }
    }
    n100 = flat-sequence {
      tunnel: w28 -> [w45]
      tunnel: w27 -> [w44]
      tunnel: w21 -> [w43]
      tunnel: [w45] -> w24
      tunnel: [w44] -> w23
      tunnel: [w40] -> w22
      tunnel: [w39] -> w20
      tunnel: w19 -> [w38]
      tunnel: [w47] -> w26
      tunnel: [w48] -> w25
      tunnel: w24 -> [w48]
      tunnel: w23 -> [w47]
      tunnel: w22 -> [w46]
      frame #0 {
        n101 = Tick Count (ms)() -> (millisecond timer value=w42:u32)
        n102 = Subtract(x=w42, y=w43) -> (x-y=w40:u32)
        n103 = Greater?(x=w40, y=w38) -> (0:w41:bool)
        n104 = Select(t=w40, s=w41, f=w38) -> (s? t:f=w39:u32)
        "loop max (ms)" <- w39
      }
      frame #1 {
        "loop time (ms)" <- w46
      }
    }
  }
  n105 = flat-sequence {
    frame #0 {
      n106 = call "ZeroMQ_PUBGS.vi"() -> ()  [unwired: 12 in]
      n107 = call "ZeroMQ_GS.vi"() -> ()  [unwired: 12 in]
      n108 = call "ServerTCPIP_Autoguider2016.vi"() -> ()  [unwired: 12 in]
    }
  }
  n109 = call-dynamic "End.vi"("error in (no error)"=w11, "S4ACS_GUI in"=w14) -> ("error out"=w12:errorcluster)  [unwired: 8 in, 1 out]
  n110 = flat-sequence {
    tunnel: w12 -> [w285]
    tunnel: [w285] -> w3
    frame #0 {
      w284 = FALSE ("ICS connection")
      n111 = local write "AG connection"(w284) -> ()
      n112 = local write "ICS connection"(w284) -> ()
      n113 = local write "GMIR status"(w284) -> ()
      n114 = local write "GFOC status"(w284) -> ()
    }
  }
  n115 = flat-sequence {
    tunnel: w3 -> [w286]
    tunnel: [w286] -> w2
    frame #0 {
      n116 = Stop() -> ()  [unwired: 1 in]
    }
  }
  "error out" <- w2
  "GUI version" <- w1
